vi "Update Vertical Scale.vi"(8 "error in (no error)":errorcluster, 9 "Volts per Division (V)":dbl, 10 "Channel Name":string, 11 "Test Scope in":refnum<class "Test Scope.lvclass">) -> (0 "error out":errorcluster, 3 "Test Scope out":refnum<class "Test Scope.lvclass">)   [LabVIEW 2015, in "Test Scope.lvclass"]
uses:
  Test Scope.lvclass
  Test Scope.lvclass/Test Scope.ctl
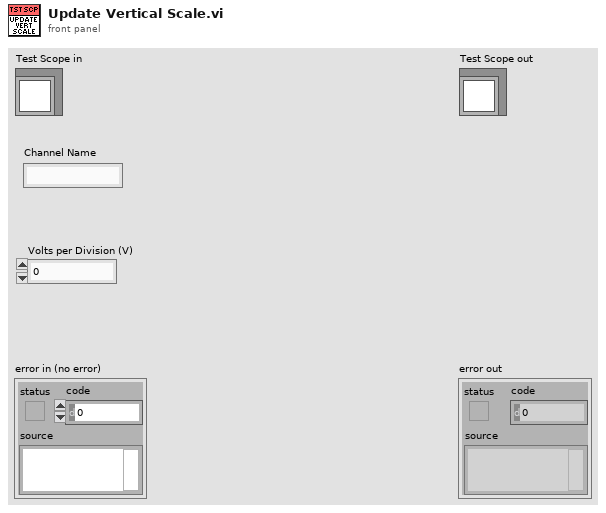
[diagram p1: front panel]
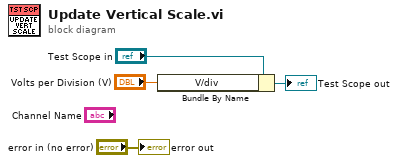
[diagram p0: block diagram]
diagram:
  n1 = Bundle By Name(cluster="Test Scope in", "V/div"="Volts per Division (V)") -> (→"Test Scope out":refnum<class "Test Scope.lvclass">)
  "error out" <- "error in (no error)"
